vi "simple_insert.vi"(8 "error in (no error)":errorcluster, 9 "Value":dbl, 10 "path table:column":string, 11 "Data.PG in":refnum<class "Data.PG.lvclass">) -> (0 "error out":errorcluster, 3 "Data.PG out":refnum<class "Data.PG.lvclass">)   [LabVIEW 2020, in "Data.PG.lvclass"]
uses:
  Data.PG.lvclass
  Data/Typedefs/Operation--enum.ctl
  Data.PG.lvclass/Data.PG.ctl
  <vilib>/JDP Science/PostgreSQL Library/Result/PQ Result.lvclass/PQ Result.ctl
  <vilib>/JDP Science/PostgreSQL Library/Connection/Execute Command (2D string results).vi
  <vilib>/JDP Science/PostgreSQL Library/Result/Clear.vi
  <vilib>/JDP Science/PostgreSQL Library/Connection/Execute Command (Result).vi
  <vilib>/JDP Science/PostgreSQL Library/Connection/Execute (Return first result with rows).vi
  <vilib>/JDP Science/PostgreSQL Library/Connection/Single Command with parameters.vi
  <vilib>/JDP Science/PostgreSQL Library/Result/Get all results as 2D strings array.vi
  <vilib>/JDP Science/PostgreSQL Library/Connection/PQ Connection.lvclass
  Data/Data.lvclass
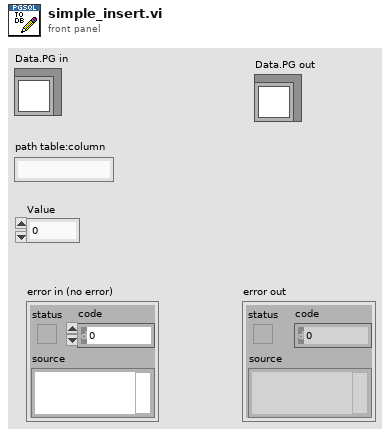
[diagram p1: front panel]
types:
  T1 = typedef "Data.lvclass/Operation--enum.ctl" = enum16{"Read", "Write", "Write + Append"}
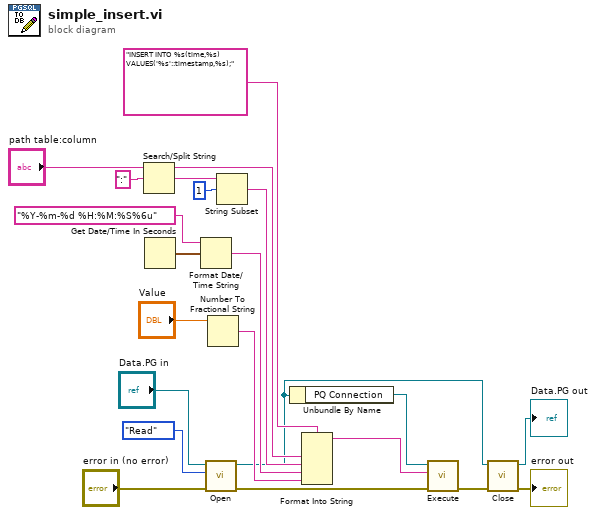
[diagram p0: block diagram]
diagram:
  n1 = Search/Split String(string="path table:column", search string/char (-)=":") -> (substring before match=w19:string, match + rest of string=w18:string)  [unwired: 1 in, 1 out]
  n2 = Get Date/Time In Seconds() -> (seconds since 1Jan1904=w13:timestamp)
  n3 = Format Date/Time String(time format string (%c)="%Y-%m-%d %H:%M:%S%6u", seconds (now)=w13) -> (date/time string=w14:string)  [unwired: 1 in]
  n4 = call-dynamic "Open.vi"("error in (no error)"="error in (no error)", "Operation"=Operation--enum."Read", "Data.PG in"="Data.PG in") -> ("error out"=w7:errorcluster, "Data.PG out"=w2:refnum<class "Data.PG.lvclass">)  [unwired: 7 in]
  n5 = Number To Fractional String(number="Value") -> (F-format string=w11:string)  [unwired: 3 in]
  n6 = String Subset(string=w18, offset (0)=1) -> (substring=w16:string)  [unwired: 1 in]
  n7 = Unbundle By Name(w2) -> ("PQ Connection"=w1:refnum<class "PQ Connection.lvclass">)
  n8 = Format Into String(format string="INSERT INTO %s(time,%s) VALUES('%s'::timestamp,%s);", w19, w16, w14, w11) -> (resulting string=w3:string)  [unwired: 2 in, 1 out]
  n9 = call-poly <vilib>:"Execute.vi"("error in (no error)"=w7, "SQL"=w3, "PQ Connection in"=w1) -> ("error out"=w6:errorcluster)  [unwired: 5 in, 3 out]
  n10 = call-dynamic "Close.vi"("error in (no error)"=w6, "Data.PG in"=w2) -> ("error out"=→"error out":errorcluster, "Data.PG out"=→"Data.PG out":refnum<class "Data.PG.lvclass">)  [unwired: 8 in]
